vi "题目1.vi"() -> ()   [LabVIEW 2017]
panel:
  out "7（X0=10,dx=2,Y）多条曲线":cluster{i32, i32, cluster{dbl[]}[]}(graph)
  out "6（X0=10,dx=2,Y）多条曲线":cluster{i32, i32, dbl[][]}(graph)
  out "5（X0=10,dx=2,Y）多条曲线":cluster{i32, i32, dbl[]}[](graph)
  out "4（X0=10,dx=2,Y）单条曲线":cluster{i32, i32, dbl[]}(graph)
  out "3（Y）多条曲线":cluster{dbl[]}[](graph)
  out "2（Y）多条曲线":dbl[][](graph)
  out "1（Y）单条曲线":dbl[](graph)
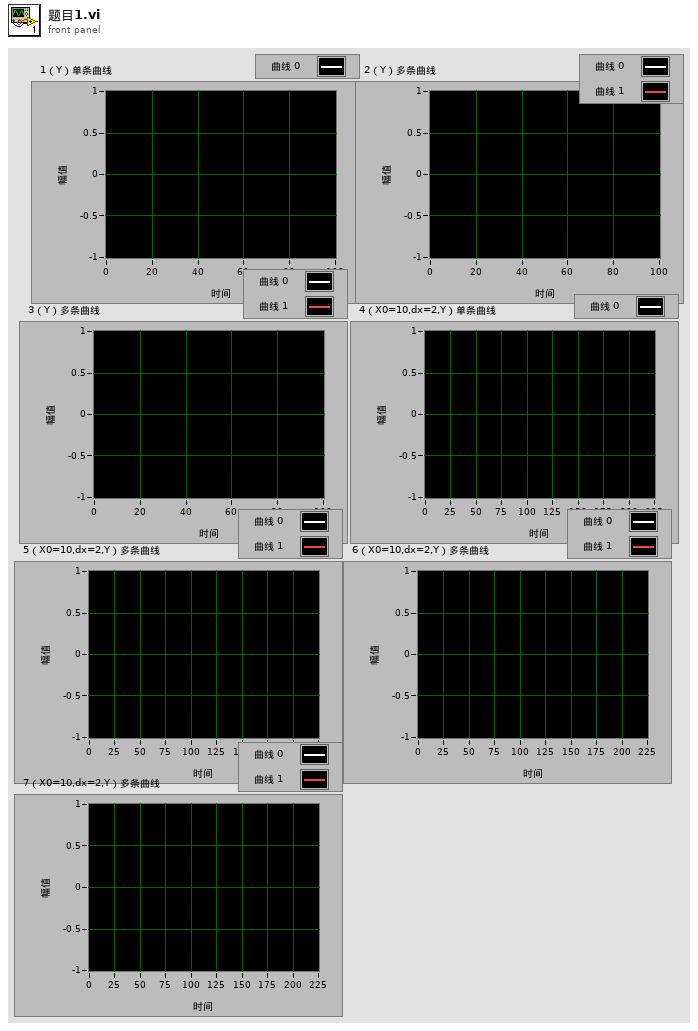
[diagram p1: front panel]
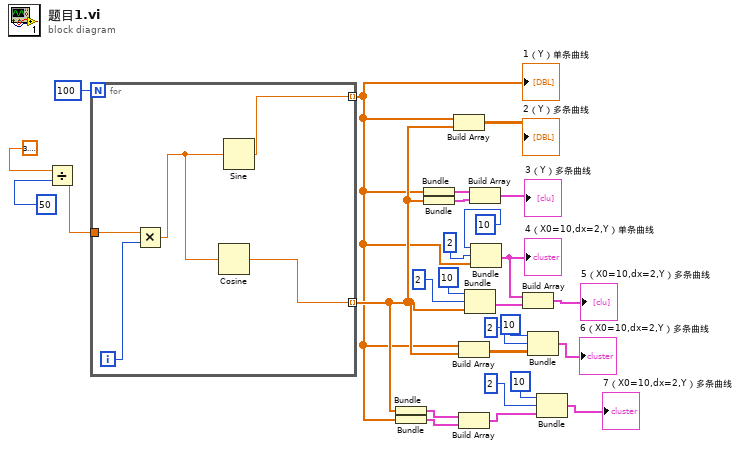
[diagram p0: block diagram]
diagram:
  n1 = Divide(x=3.141592653589793, y=50) -> (x/y=w24:dbl)
  n2 = for {
    N: 100 -> [_]
    tunnel: w24 -> [w32]
    tunnel: [w29] -> w5 mode=indexing
    tunnel: [w28] -> w6 mode=indexing
    i -> [w31]
    n3 = Multiply(x=w32, y=w31) -> (x*y=w30:dbl)
    n4 = Cosine(x=w30) -> (cos(x)=w28:dbl)
    n5 = Sine(x=w30) -> (sin(x)=w29:dbl)
  }
  "1（Y）单条曲线" <- w5
  n6 = Bundle(w6) -> (w4:cluster{dbl[]})  [unwired: 1 in]
  n7 = Bundle(w5) -> (w3:cluster{dbl[]})  [unwired: 1 in]
  n8 = Bundle(w5) -> (w22:cluster{dbl[]})  [unwired: 1 in]
  n9 = Bundle(w6) -> (w21:cluster{dbl[]})  [unwired: 1 in]
  n10 = Build Array(w5, w6) -> (→"2（Y）多条曲线":dbl[][])
  n11 = Build Array(w5, w6) -> (w8:dbl[][])
  n12 = Build Array(w4, w3) -> (w2:cluster{dbl[]}[])
  n13 = Bundle(10, 2, w6) -> (w14:cluster{i32, i32, dbl[]})  [unwired: 1 in]
  n14 = Build Array(w22, w21) -> (→"3（Y）多条曲线":cluster{dbl[]}[])
  n15 = Bundle(10, 2, w5) -> (w15:cluster{i32, i32, dbl[]})  [unwired: 1 in]
  "4（X0=10,dx=2,Y）单条曲线" <- w15
  n16 = Build Array(w15, w14) -> (→"5（X0=10,dx=2,Y）多条曲线":cluster{i32, i32, dbl[]}[])
  n17 = Bundle(10, 2, w8) -> (→"6（X0=10,dx=2,Y）多条曲线":cluster{i32, i32, dbl[][]})  [unwired: 1 in]
  n18 = Bundle(10, 2, w2) -> (→"7（X0=10,dx=2,Y）多条曲线":cluster{i32, i32, cluster{dbl[]}[]})  [unwired: 1 in]
